vi "SDCP SMF Receiver and Trasmitter - Live Plot - Backup.vi"() -> ()   [LabVIEW 2020]
uses:
  Typedefs/SDCP - Standard Message Frame Parameters - FGV - commands.ctl
  Typedefs/SDCP - Serial Port Control - Commands.ctl
panel:
  out "Active Plot Names":string[](array[string])
  out "Value":dbl
  out "Time (ms)":dbl
  in  "Cursor Parameter":string(combo)
  out "Instantaeneous data":T1(array[cluster])
  in  "Time span (ms)":dbl
  in  "Channel 8 enable":bool
  in  "Channel 7 enable":bool
  in  "Channel 6 enable":bool
  in  "Channel 5 enable":bool
  in  "Channel 4 enable":bool
  in  "Channel 3 enable":bool
  in  "Channel 2 enable":bool
  in  "Channel 1 enable":bool
  in  "Channel 8 parameter":string(combo)
  in  "Channel 7 parameter":string(combo)
  in  "Channel 6 parameter":string(combo)
  in  "Channel 5 parameter":string(combo)
  in  "Channel 4 parameter":string(combo)
  in  "Channel 3 parameter":string(combo)
  in  "Channel 2 parameter":string(combo)
  in  "Channel 1 parameter":string(combo)
  in  "Plot file path":path
  out "Live Plot":T2(graph)
  out "Time (ms)":u32
  in  "Stop Application":bool
  in  "Trace file path":path
  in  "Baud rate":u32=9600
  in  "COM Port":refnum<visa-resource-name>
  in  "Parameter file path":path=path "E:/Projects/System Diagnostics and Control Protocol/SDCP_LabVIEW/Parameter Files/Motion_Processing.param"
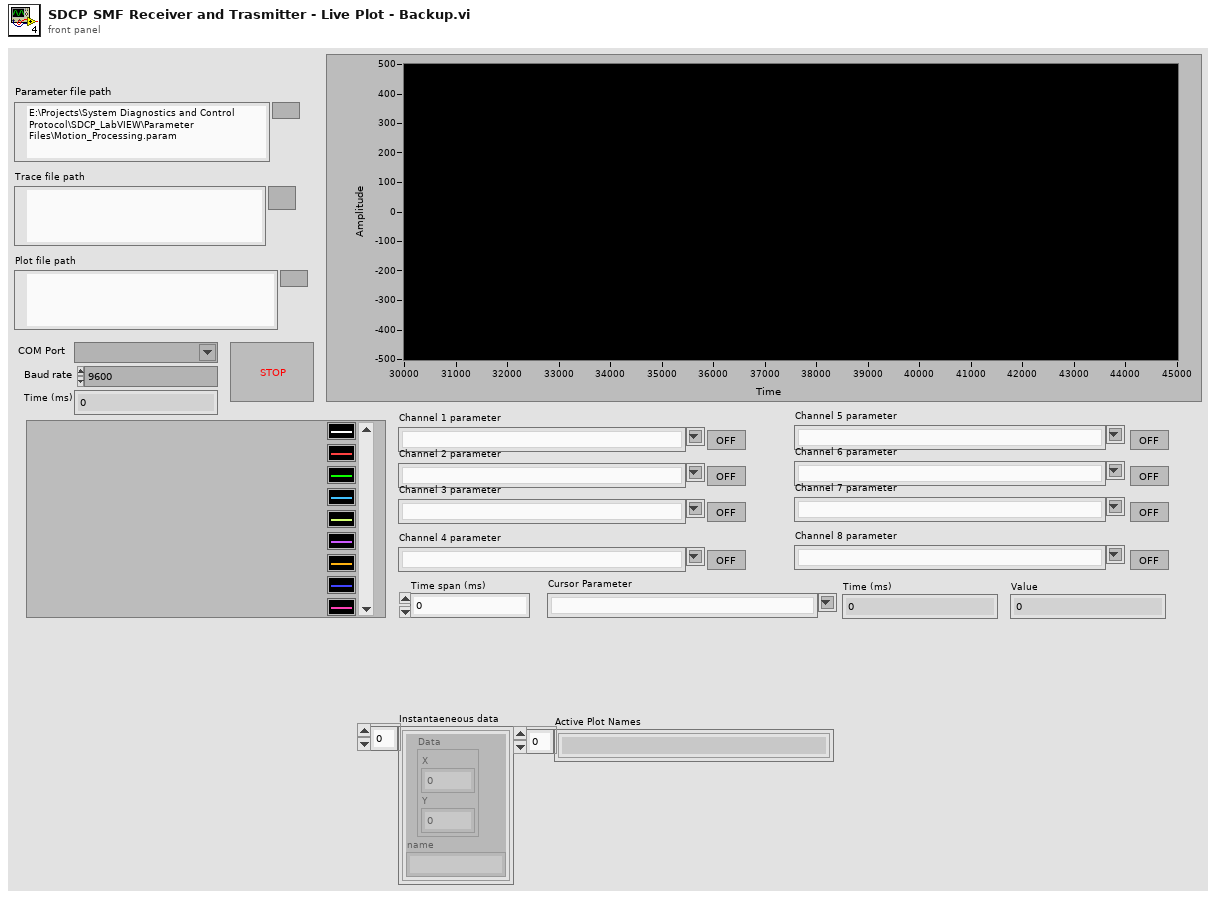
[diagram p1: front panel]
types:
  T1 = cluster{"Data":cluster{"X":dbl, "Y":dbl}, "name":string}[]
  T2 = cluster{"Plot data":cluster{"X":dbl, "Y":dbl}[]}[]
  T3 = typedef "SDCP - Serial Port Control - Commands.ctl" = enum16{"Open", "Read", "Write", "Get instance", "Close"}
  T4 = cluster{"data bytes":u8[], "Time (ms)":u32, "Direction":string}
  T5 = typedef "SDCP - Standard Message Frame Parameters - FGV - commands.ctl" = enum16{"Write descriptors", "Read descriptors", "Read values", "Load parameters from file", "Write values", "Read all descriptors"}
  T6 = typedef "SDCP - SMF parameter descriptors.ctl" = cluster{"Frame name":string, "Frame ID":i32, "Data type":string, "Start Position":i32, "Length":i32, "Factor":dbl, "Offset":dbl, "Parameter name":string, "Value":string}
  T7 = cluster{"name":string, "Data":cluster{"X":dbl, "Y":dbl}[]}
  T8 = cluster{"name":string, "Data":cluster{"X":dbl, "Y":dbl}[]}[]
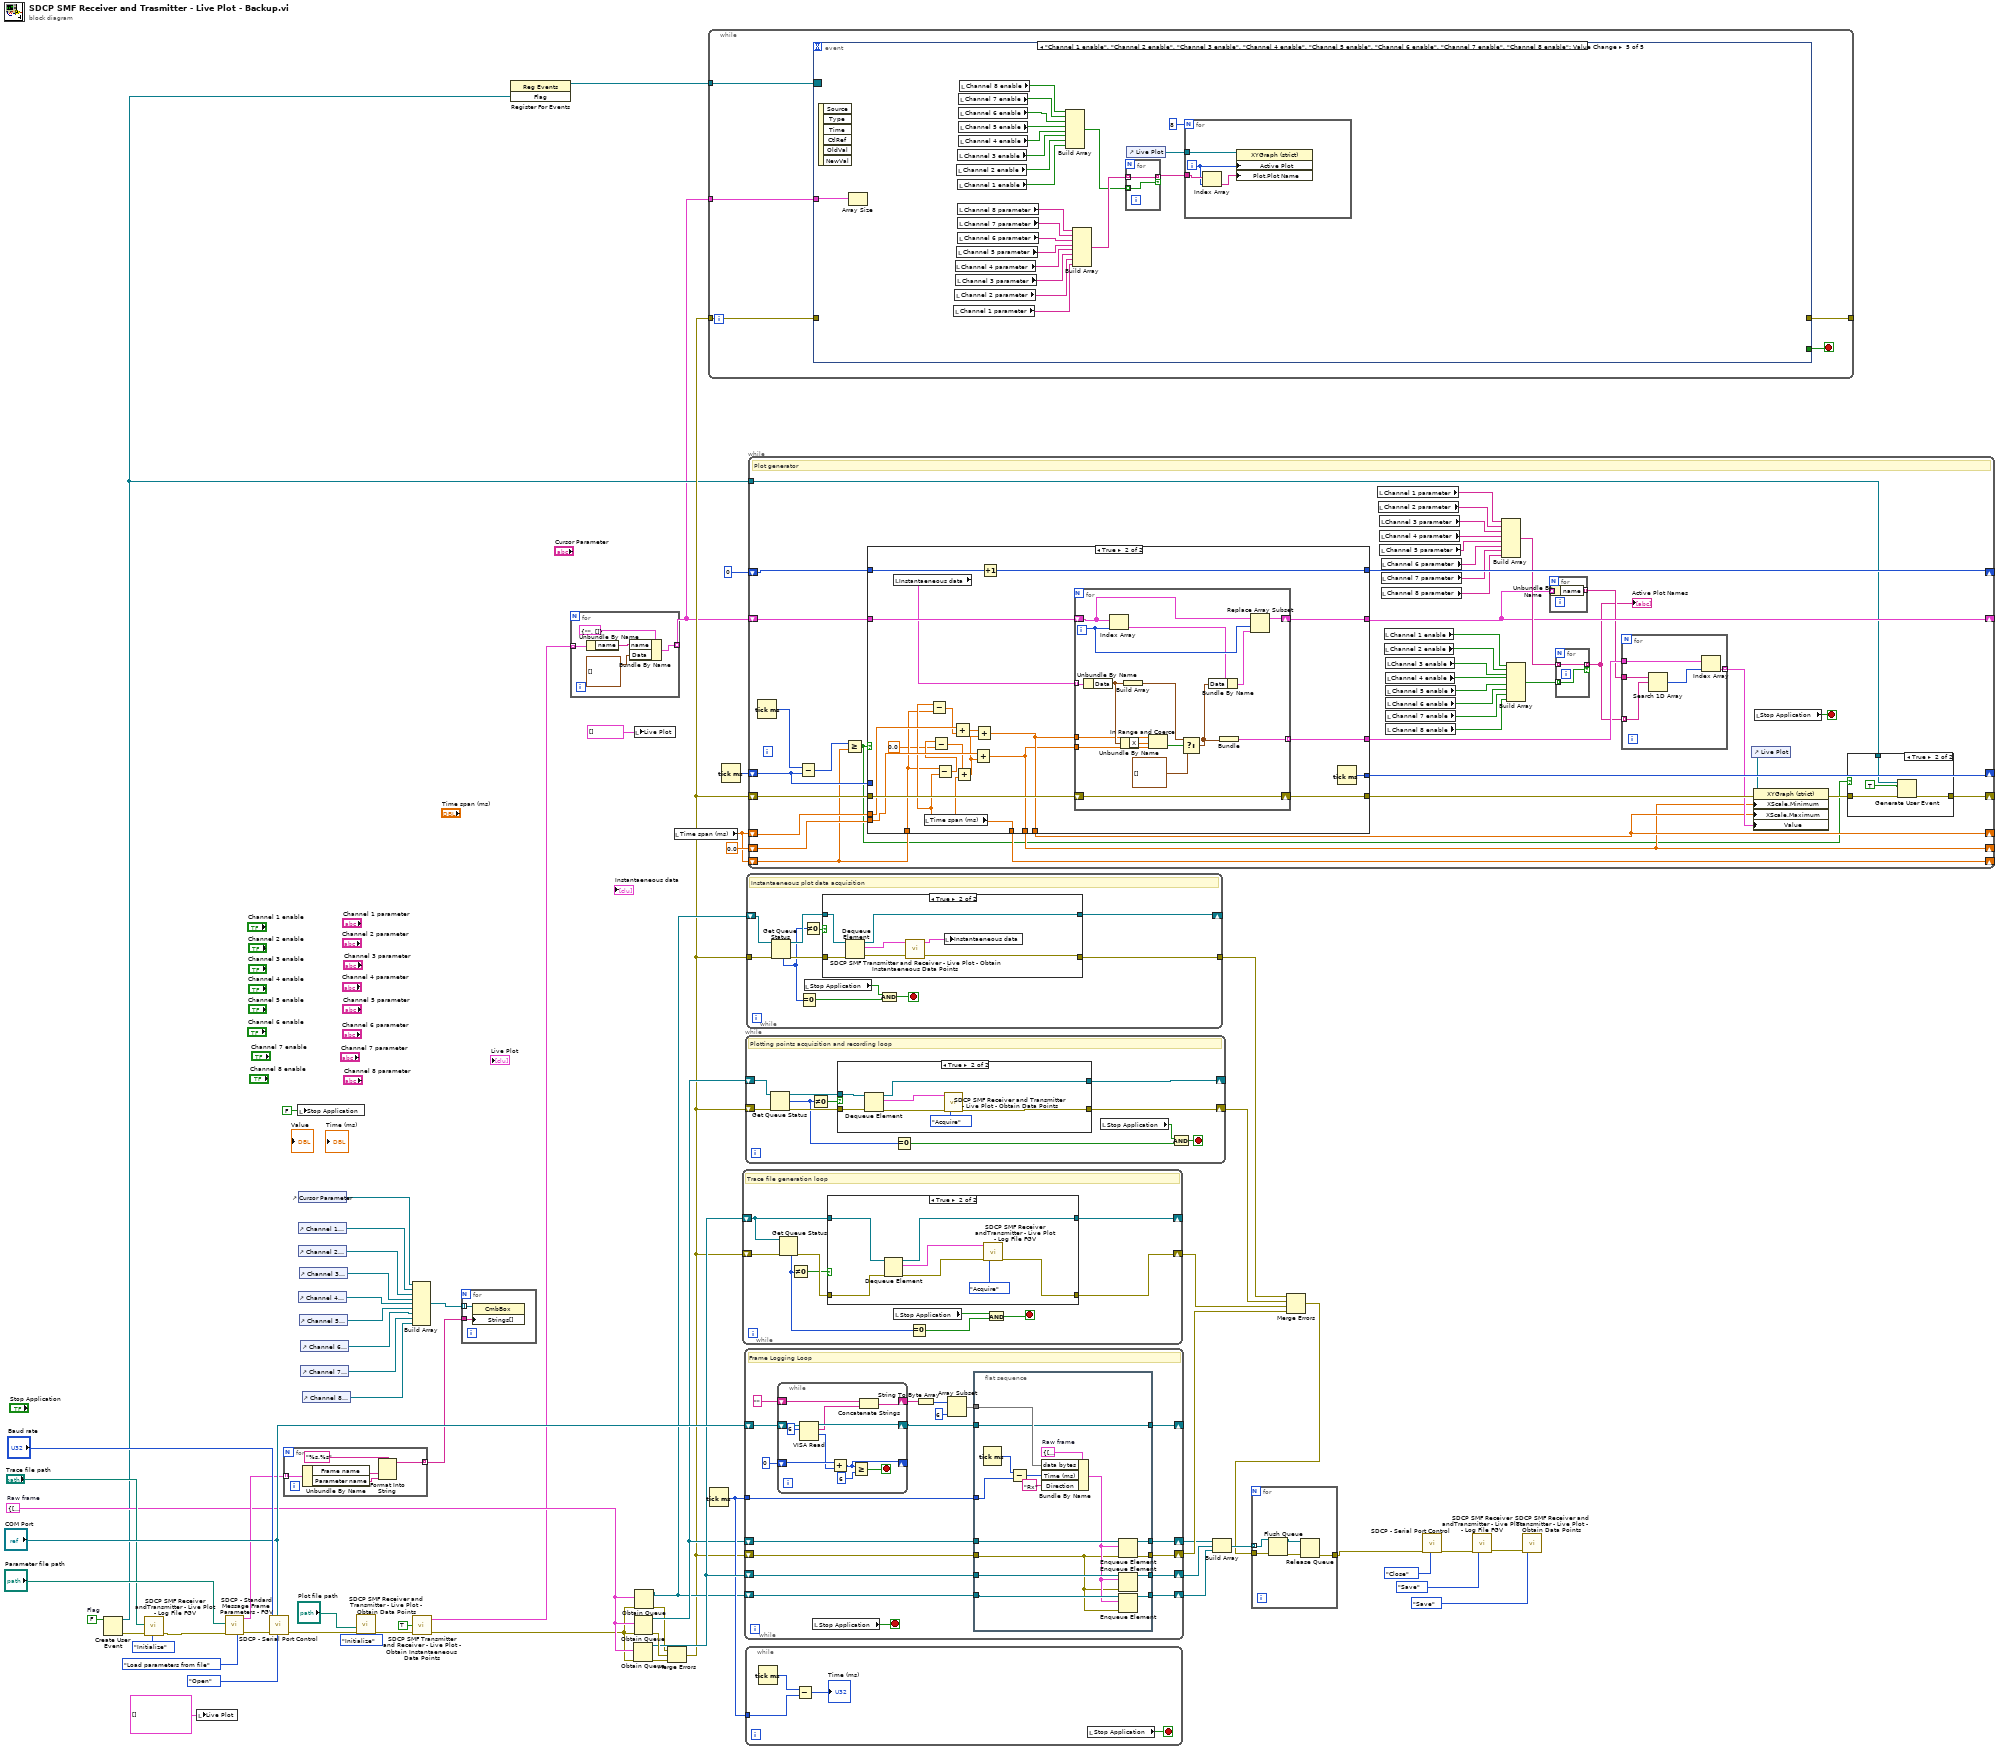
[diagram p0: block diagram]
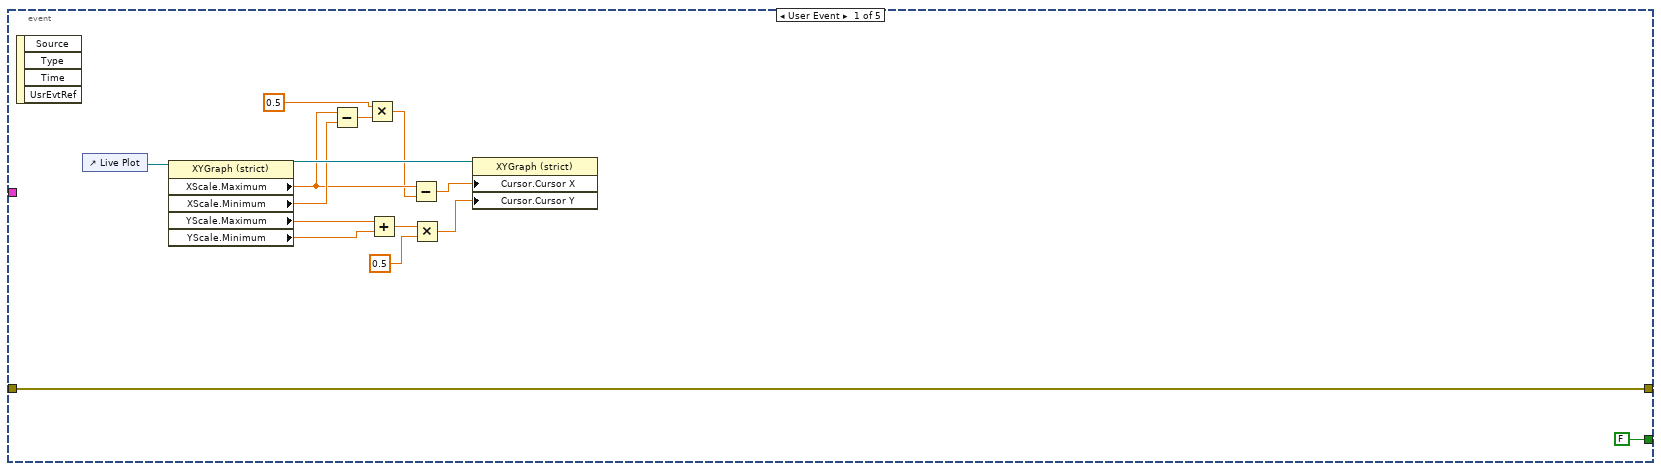
[diagram p2: hidden frame]
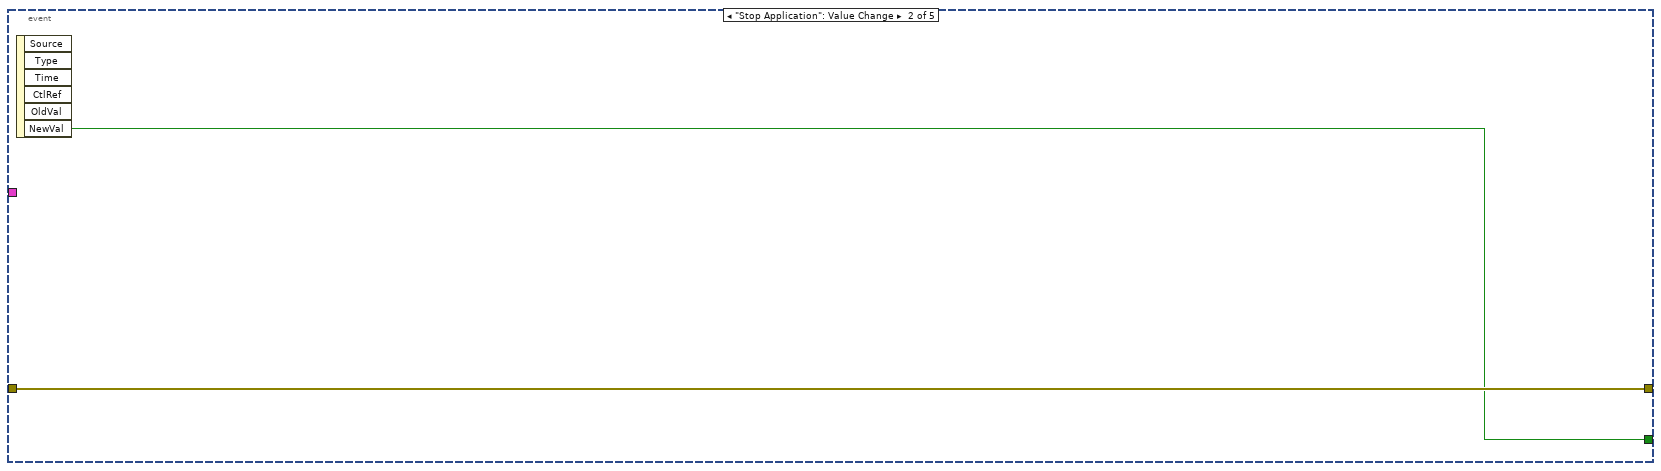
[diagram p3: hidden frame]
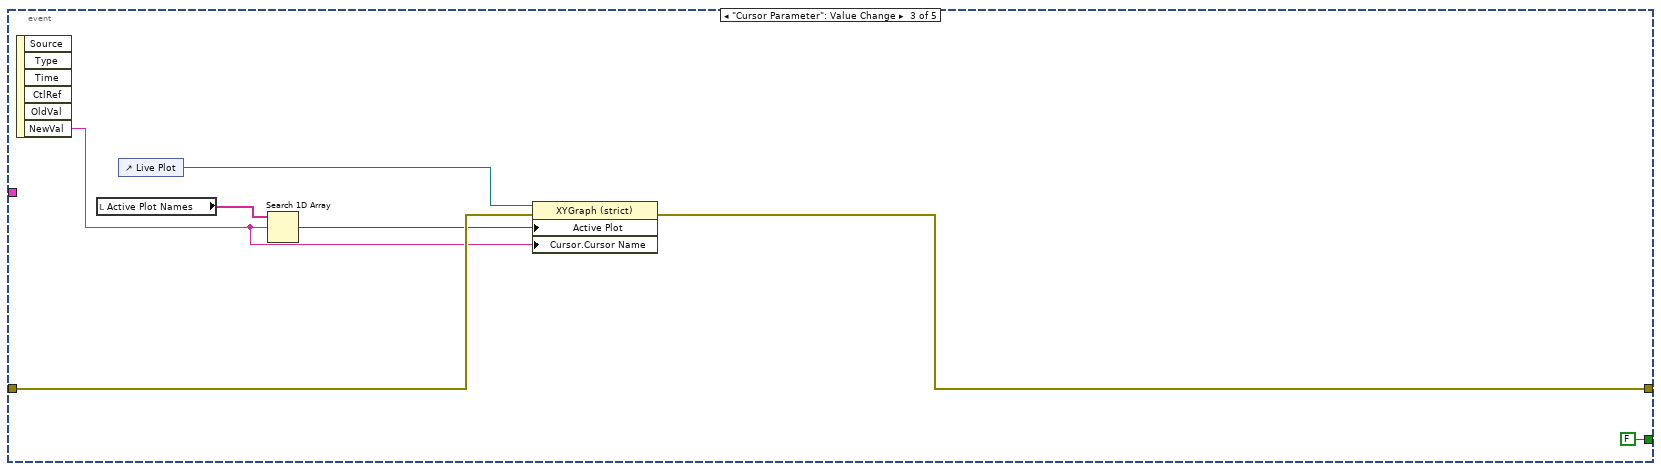
[diagram p4: hidden frame]
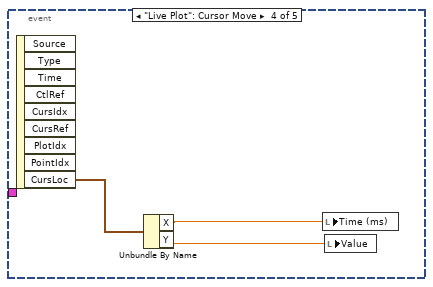
[diagram p5: hidden frame]
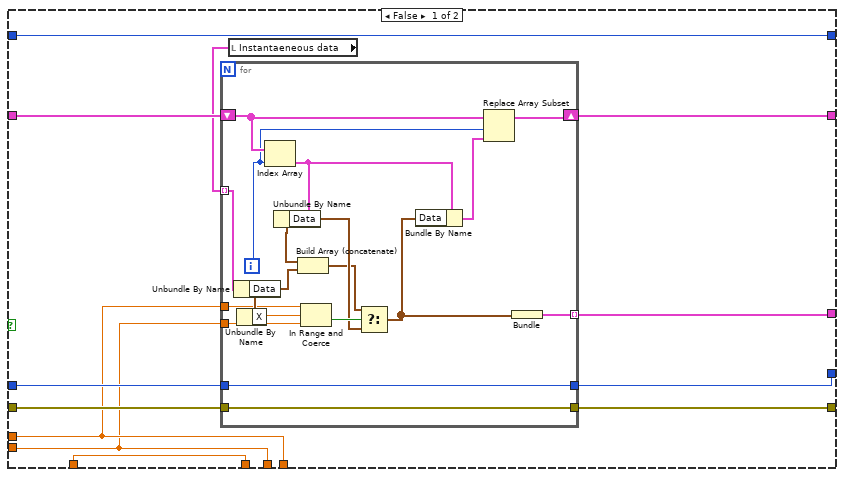
[diagram p7: hidden frame]
diagram:
  w4 = FALSE  # Flag
  w28 = T4 {"data bytes"=[], "Time (ms)"=0, "Direction"=""}  # Raw frame
  n1 = Create User Event(user event datatype=w4) -> (user event=w2:refnum<user-event>, error out=w5:errorcluster)  [unwired: 1 in]
  n2 = call "SDCP SMF Receiver andTransmitter - Live Plot - Log File FGV.vi"("error in (no error)"=w5, "Command"=enum16{"Initialize", "Acquire", "Save"}."Initialize", "Trace file path"="Trace file path") -> ("error out"=w46:errorcluster)  [unwired: 4 in]
  n3 = local write "Live Plot"(T2 [] ("Live Plot")) -> ()
  n4 = call "SDCP - Standard Message Frame Parameters - FGV.vi"("Parameter file path"="Parameter file path", "error in (no error)"=w46, "Command"=SDCP_-_Standard_Message_Frame_Parameters_-_FGV_-_commands."Load parameters from file") -> ("SMF Parameters descriptors out"=w41:T6[], "error out"=w62:errorcluster)  [unwired: 4 in]
  n5 = call "SDCP - Serial Port Control.vi"("Command"=SDCP_-_Serial_Port_Control_-_Commands."Open", "VISA resource name"="COM Port", "error in (no error)"=w62, "Baud rate"="Baud rate") -> ("error out"=w30:errorcluster)  [unwired: 4 in, 3 out]
  n6 = for {
    tunnel: w41 -> [w69] mode=indexing
    tunnel: [w65] -> w31 mode=indexing
    n7 = Unbundle By Name(w69) -> ("Frame name"=w67:string, "Parameter name"=w66:string)
    n8 = Format Into String(format string="%s.%s", w67, w66) -> (resulting string=w65:string)  [unwired: 2 in, 1 out]
  }
  n9 = local write "Stop Application"(FALSE ("Stop Application")) -> ()
  n10 = control-ref of="Cursor Parameter"() -> (w7:refnum<vi>)
  n11 = control-ref of="Channel 1 parameter"() -> (w40:refnum<vi>)
  n12 = control-ref of="Channel 2 parameter"() -> (w39:refnum<vi>)
  n13 = control-ref of="Channel 4 parameter"() -> (w37:refnum<vi>)
  n14 = control-ref of="Channel 3 parameter"() -> (w38:refnum<vi>)
  n15 = control-ref of="Channel 5 parameter"() -> (w36:refnum<vi>)
  n16 = control-ref of="Channel 6 parameter"() -> (w35:refnum<vi>)
  n17 = control-ref of="Channel 7 parameter"() -> (w34:refnum<vi>)
  n18 = control-ref of="Channel 8 parameter"() -> (w33:refnum<vi>)
  n19 = call "SDCP SMF Receiver and Transmitter - Live Plot - Obtain Data Points.vi"("error in (no error)"=w30, "Plot file path"="Plot file path", "Command"=enum16{"Initialize", "Acquire", "Save"}."Initialize") -> ("error out"=w17:errorcluster)  [unwired: 4 in]
  n20 = Build Array(w7, w40, w39, w38, w37, w36, w35, w34, w33) -> (w32:refnum<vi>[])
  n21 = call "SDCP SMF Transmitter and Receiver - Live Plot - Obtain Instantaeneous Data Points.vi"("error in (no error)"=w17, "Initialize ?"=TRUE) -> ("error out"=w16:errorcluster, "Instantaeneous data"=w13:T1)  [unwired: 2 in]
  n22 = for {
    tunnel: w32 -> [w71] mode=indexing
    tunnel: w31 -> [w70]
    n23 = property class="CmbBox"(reference=w71, "Strings[]"=w70) -> ()  [unwired: 1 in, 2 out]
  }
  n24 = register-events(w2) -> (reference out=w3:refnum<event-registration>)  [unwired: 2 in, 1 out]
  n25 = for {
    tunnel: w13 -> [w76] mode=indexing
    tunnel: [w73] -> w1 mode=indexing
    n26 = Unbundle By Name(w76) -> ("name"=w74:string)
    n27 = Bundle By Name(cluster=T7 {"name"="", "Data"=[]}, "name"=w74, "Data"=cluster{"X":dbl, "Y":dbl}[] []) -> (w73:T7)
  }
  n28 = Obtain Queue(element data type=w28, error in (no error)=w16) -> (queue out=w56:refnum<queue>, error out=w57:errorcluster)  [unwired: 3 in, 1 out]
  n29 = local write "Live Plot"(cluster{"Data":cluster{"X":dbl, "Y":dbl}[]}[] []) -> ()
  n30 = Obtain Queue(element data type=w28, error in (no error)=w16) -> (queue out=w47:refnum<queue>, error out=w58:errorcluster)  [unwired: 3 in, 1 out]
  n31 = Obtain Queue(element data type=w28, error in (no error)=w16) -> (queue out=w19:refnum<queue>, error out=w27:errorcluster)  [unwired: 3 in, 1 out]
  n32 = Merge Errors(w27, w58, w57) -> (w6:errorcluster)
  n33 = local read "Time span (ms)"() -> (w8:dbl)
  n34 = while {
    tunnel: w6 -> [w81]
    tunnel: [w80] -> _
    tunnel: w3 -> [w78]
    tunnel: w1 -> [w77]
    stop <- w79 stop-if-true
    n35 = event shown="[4] \"Channel 1 enable\", \"Channel 2 enable\", \"Channel 3 enable\", \"Channel 4 enable\", \"Channel 5 enable\", \"Channel 6 enable\", \"Channel 7 enable\", \"Channel 8 enable\": Value Change" {
      selector: w78 -> [_ _ _ _ _]
      dyn-events: _ -> [_ _ _ _ _]
      timeout: _ -> [_ _ _ _ _]
      tunnel: w81 -> [w96 w98 w104 _ _]
      tunnel: [w96 w98 w100 _ _] -> w80
      tunnel: [FALSE w97 FALSE ("NewVal") _ _] -> w79
      tunnel: w77 -> [_ _ _ _ w110]
      event User Event {
        n36 = event-data() -> ()  [unwired: 1 in, 4 out]
        n37 = control-ref of="Live Plot"() -> (w94:refnum<vi>)
        n38 = property class="XYGraph (strict)"(reference=w94) -> (reference out=w89:refnum<vi>, "XScale.Maximum"=w86:dbl, "XScale.Minimum"=w87:dbl, "YScale.Maximum"=w93:dbl, "YScale.Minimum"=w92:dbl)  [unwired: 1 in, 1 out]
        n39 = Subtract(x=w86, y=w87) -> (x-y=w85:dbl)
        n40 = Multiply(x=0.5, y=w85) -> (x*y=w83:dbl)
        n41 = Add(x=w93, y=w92) -> (x+y=w91:dbl)
        n42 = Subtract(x=w86, y=w83) -> (x-y=w82:dbl)
        n43 = Multiply(x=w91, y=0.5) -> (x*y=w88:dbl)
        n44 = property class="XYGraph (strict)"(reference=w89, "Cursor.Cursor X"=w82, "Cursor.Cursor Y"=w88) -> ()  [unwired: 1 in, 2 out]
      }
      event "Stop Application": Value Change {
        n45 = event-data() -> ("NewVal"=w97:bool)  [unwired: 1 in, 5 out]
      }
      event "Cursor Parameter": Value Change {
        n46 = event-data() -> ("NewVal"=w101:string)  [unwired: 1 in, 5 out]
        n47 = local read "Active Plot Names"() -> (w99:string[])
        n48 = control-ref of="Live Plot"() -> (w103:refnum<vi>)
        n49 = Search 1D Array(1D array=w99, element=w101) -> (index of element=w102:i32)  [unwired: 1 in]
        n50 = property class="XYGraph (strict)"(reference=w103, error in=w104, "Active Plot"=w102, "Cursor.Cursor Name"=w101) -> (error out=w100:errorcluster)  [unwired: 1 out]
      }
      event "Live Plot": Cursor Move {
        n51 = event-data() -> ("CursLoc"=w108:cluster{"X":dbl, "Y":dbl})  [unwired: 1 in, 8 out]
        n52 = Unbundle By Name(w108) -> ("X"=w107:dbl, "Y"=w106:dbl)
        n53 = local write "Time (ms)"(w107) -> ()
        n54 = local write "Value"(w106) -> ()
      }
      event "Channel 1 enable", "Channel 2 enable", "Channel 3 enable", "Channel 4 enable", "Channel 5 enable", "Channel 6 enable", "Channel 7 enable", "Channel 8 enable": Value Change {
        n55 = event-data() -> ()  [unwired: 1 in, 6 out]
        n56 = Array Size(array=w110) -> ()  [unwired: 1 out]
        n57 = local read "Channel 1 parameter"() -> (w115:string)
        n58 = local read "Channel 2 parameter"() -> (w116:string)
        n59 = local read "Channel 4 parameter"() -> (w118:string)
        n60 = local read "Channel 3 parameter"() -> (w117:string)
        n61 = local read "Channel 2 enable"() -> (w124:bool)
        n62 = local read "Channel 5 parameter"() -> (w119:string)
        n63 = local read "Channel 3 enable"() -> (w125:bool)
        n64 = local read "Channel 1 enable"() -> (w123:bool)
        n65 = local read "Channel 8 parameter"() -> (w122:string)
        n66 = local read "Channel 7 parameter"() -> (w121:string)
        n67 = local read "Channel 6 parameter"() -> (w120:string)
        n68 = local read "Channel 7 enable"() -> (w129:bool)
        n69 = local read "Channel 6 enable"() -> (w128:bool)
        n70 = local read "Channel 5 enable"() -> (w127:bool)
        n71 = local read "Channel 4 enable"() -> (w126:bool)
        n72 = local read "Channel 8 enable"() -> (w130:bool)
        n73 = Build Array(w130, w129, w128, w127, w126, w125, w124, w123) -> (w113:bool[])
        n74 = Build Array(w122, w121, w120, w119, w118, w117, w116, w115) -> (w114:string[])
        n75 = for {
          tunnel: w114 -> [w136] mode=indexing
          tunnel: w113 -> [w135] mode=indexing
          tunnel: [w136] -> w111 mode=indexing if=w135
        }
        n76 = control-ref of="Live Plot"() -> (w112:refnum<vi>)
        n77 = for {
          N: 8 -> [_]
          tunnel: w112 -> [w134]
          tunnel: w111 -> [w133]
          i -> [w132]
          n78 = Index Array(array=w133, index=w132) -> (element=w131:string)
          n79 = property class="XYGraph (strict)"(reference=w134, "Active Plot"=w132, "Plot.Plot Name"=w131) -> ()  [unwired: 1 in, 2 out]
        }
      }
    }
  }
  n80 = Tick Count (ms)() -> (millisecond timer value=w48:u32)
  n81 = Tick Count (ms)() -> (millisecond timer value=w14:u32)
  n82 = while {
    shift-right: [w144] -> w50
    shift-left: w6 -> [w146]
    shift-right: [w143] -> _
    shift-left: w56 -> [w145]
    stop <- w139 stop-if-true
    # "Trace file generation loop"
    n83 = Get Queue Status(queue=w145, error in (no error)=w146) -> (error out=w142:errorcluster, # elements in queue=w138:i32)  [unwired: 1 in, 6 out]
    n84 = Not Equal To 0?(x=w138) -> (x != 0?=w141:bool)
    n85 = case shown="True" w141 {
      tunnel: w142 -> [w148 w153]
      tunnel: [w148 w155] -> w144
      tunnel: w145 -> [w147 w151]
      tunnel: [w147 w150] -> w143
      frame False {
      }
      frame True {
        n86 = Dequeue Element(queue=w151, error in (no error)=w153) -> (queue out=w150:refnum<queue>, element=w149:T4, error out=w152:errorcluster)  [unwired: 1 in, 1 out]
        n87 = call "SDCP SMF Receiver andTransmitter - Live Plot - Log File FGV.vi"("error in (no error)"=w152, "Command"=enum16{"Initialize", "Acquire", "Save"}."Acquire", "Raw frame"=w149) -> ("error out"=w155:errorcluster)  [unwired: 4 in]
      }
    }
    n88 = local read "Stop Application"() -> (w140:bool)
    n89 = Equal To 0?(x=w138) -> (x = 0?=w137:bool)
    n90 = And(x=w140, y=w137) -> (x .and. y?=w139:bool)
  }
  n91 = while {
    tunnel: w48 -> [w167]
    shift-right: [w163] -> _
    shift-left: "COM Port" -> [w174]
    shift-right: [w165] -> w49
    shift-left: w6 -> [w166]
    shift-right: [w161] -> w25
    shift-left: w47 -> [w162]
    shift-right: [w159] -> w24
    shift-left: w56 -> [w160]
    shift-right: [w156] -> w23
    shift-left: w19 -> [w157]
    stop <- w158 stop-if-true
    # "Frame Logging Loop"
    n92 = while {
      shift-right: [w200] -> w164
      shift-left: w174 -> [w201]
      shift-right: [w192] -> w171
      shift-left: "" -> [w194]
      shift-right: [w196] -> _
      shift-left: 0 -> [w199]
      stop <- w195 stop-if-true
      n93 = VISA Read(VISA resource name=w201, byte count=u32 6) -> (VISA resource name out=w200:refnum<visa-resource-name>, read buffer=w193:string, return count=w198:u32)  [unwired: 1 in, 1 out]
      n94 = Add(x=w199, y=w198) -> (x+y=w196:u32)
      n95 = Greater Or Equal?(x=w196, y=u32 6) -> (x >= y?=w195:bool)
      n96 = Concatenate Strings(w194, w193) -> (w192:string)
    }
    n97 = local read "Stop Application"() -> (w158:bool)
    n98 = String To Byte Array(string=w171) -> (unsigned byte array=w170:u8[])
    n99 = Array Subset(array=w170, length=6) -> (w168:u8[])  [unwired: 1 in]
    n100 = flat-sequence {
      tunnel: w168 -> [w180]
      tunnel: w167 -> [w189]
      tunnel: w166 -> [w175]
      tunnel: [w186] -> w165
      tunnel: w164 -> [w179]
      tunnel: [w179] -> w163
      tunnel: w162 -> [w185]
      tunnel: [w184] -> w161
      tunnel: w160 -> [w183]
      tunnel: [w182] -> w159
      tunnel: w157 -> [w178]
      tunnel: [w176] -> w156
      frame #0 {
        w188 = T4 {"data bytes"=[], "Time (ms)"=0, "Direction"=""}  # Raw frame
        n101 = Tick Count (ms)() -> (millisecond timer value=w190:u32)
        n102 = Subtract(x=w190, y=w189) -> (x-y=w187:u32)
        n103 = Bundle By Name(cluster=w188, "data bytes"=w180, "Time (ms)"=w187, "Direction"="Rx") -> (w177:T4)
        n104 = Enqueue Element(queue=w185, element=w177, error in (no error)=w175) -> (queue out=w184:refnum<queue>, error out=w186:errorcluster)  [unwired: 1 in, 1 out]
        n105 = Enqueue Element(queue=w183, element=w177, error in (no error)=w175) -> (queue out=w182:refnum<queue>)  [unwired: 1 in, 2 out]
        n106 = Enqueue Element(queue=w178, element=w177, error in (no error)=w175) -> (queue out=w176:refnum<queue>)  [unwired: 1 in, 2 out]
      }
    }
  }
  n107 = while {
    shift-right: [w206] -> _
    shift-left: w47 -> [w211]
    shift-right: [w208] -> w26
    shift-left: w6 -> [w212]
    stop <- w204 stop-if-true
    # "Plotting points acquisition and recording loop"
    n108 = Get Queue Status(queue=w211, error in (no error)=w212) -> (queue out=w207:refnum<queue>, error out=w209:errorcluster, # elements in queue=w205:i32)  [unwired: 1 in, 5 out]
    n109 = Not Equal To 0?(x=w205) -> (x != 0?=w210:bool)
    n110 = case shown="True" w210 {
      tunnel: w209 -> [w214 w221]
      tunnel: [w214 w216] -> w208
      tunnel: w207 -> [w213 w220]
      tunnel: [w213 w219] -> w206
      frame False {
      }
      frame True {
        n111 = Dequeue Element(queue=w220, error in (no error)=w221) -> (queue out=w219:refnum<queue>, element=w217:T4, error out=w218:errorcluster)  [unwired: 1 in, 1 out]
        n112 = call "SDCP SMF Receiver and Transmitter - Live Plot - Obtain Data Points.vi"("error in (no error)"=w218, "Command"=enum16{"Initialize", "Acquire", "Save"}."Acquire", "Raw frame"=w217) -> ("error out"=w216:errorcluster)  [unwired: 4 in]
      }
    }
    n113 = Equal To 0?(x=w205) -> (x = 0?=w202:bool)
    n114 = local read "Stop Application"() -> (w203:bool)
    n115 = And(x=w203, y=w202) -> (x .and. y?=w204:bool)
  }
  n116 = while {
    tunnel: w48 -> [w224]
    stop <- w222 stop-if-true
    n117 = Tick Count (ms)() -> (millisecond timer value=w225:u32)
    n118 = Subtract(x=w225, y=w224) -> (x-y=→"Time (ms)":u32)
    n119 = local read "Stop Application"() -> (w222:bool)
  }
  n120 = while {
    shift-right: [w228] -> _
    shift-left: w19 -> [w235]
    tunnel: w6 -> [w236]
    tunnel: [w227] -> w18
    stop <- w231 stop-if-true
    # "Instantaeneous plot data acquisition"
    n121 = Get Queue Status(queue=w235, error in (no error)=w236) -> (queue out=w229:refnum<queue>, error out=w230:errorcluster, # elements in queue=w226:i32)  [unwired: 1 in, 5 out]
    n122 = Equal To 0?(x=w226) -> (x = 0?=w233:bool)
    n123 = Not Equal To 0?(x=w226) -> (x != 0?=w234:bool)
    n124 = local read "Stop Application"() -> (w232:bool)
    n125 = case shown="True" w234 {
      tunnel: w230 -> [w237 w245]
      tunnel: w229 -> [w238 w244]
      tunnel: [w238 w243] -> w228
      tunnel: [w237 w240] -> w227
      frame False {
      }
      frame True {
        n126 = Dequeue Element(queue=w244, error in (no error)=w245) -> (queue out=w243:refnum<queue>, element=w241:T4, error out=w242:errorcluster)  [unwired: 1 in, 1 out]
        n127 = call "SDCP SMF Transmitter and Receiver - Live Plot - Obtain Instantaeneous Data Points.vi"("error in (no error)"=w242, "Raw frame"=w241) -> ("error out"=w240:errorcluster, "Instantaeneous data"=w239:T1)  [unwired: 2 in]
        n128 = local write "Instantaeneous data"(w239) -> ()
      }
    }
    n129 = And(x=w232, y=w233) -> (x .and. y?=w231:bool)
  }
  n130 = while {
    shift-right: [w249] -> _
    shift-left: w6 -> [w286]
    shift-right: [w285] -> _
    shift-left: w14 -> [w283]
    shift-right: [w258] -> _
    shift-left: w1 -> [w284]
    shift-right: [w282] -> _
    shift-left: 0 -> [w281]
    shift-right: [w256] -> _
    shift-left: w8 -> [w255]
    shift-right: [w253] -> _
    shift-left: 0.0 -> [w254]
    shift-right: [w252] -> _
    shift-left: w8 -> [w251]
    tunnel: w2 -> [w248]
    stop <- w289 stop-if-true
    # "Plot generator"
    n131 = Tick Count (ms)() -> (millisecond timer value=w288:u32)
    n132 = Subtract(x=w288, y=w283) -> (x-y=w287:u32)
    n133 = Greater Or Equal?(x=w287, y=w251) -> (x >= y?=w247:bool)
    n134 = case shown="True" w247 {
      tunnel: w286 -> [w310 w348]
      tunnel: [w309 w349] -> w280
      tunnel: [w312 w353] -> w285
      tunnel: w284 -> [w315 w352]
      tunnel: [w311 w350] -> w258
      tunnel: w283 -> [w313 _]
      tunnel: [w307 w347] -> w260
      tunnel: w281 -> [w308 w346]
      tunnel: [w308 w345] -> w282
      tunnel: [w306 w342] -> w256
      tunnel: [w305 w341] -> w253
      tunnel: w255 -> [w306 w344]
      tunnel: w254 -> [w305 w343]
      tunnel: [w304 w339] -> w252
      tunnel: w251 -> [w304 w338]
      frame False {
        n135 = local read "Instantaeneous data"() -> (w314:T1)
        n136 = for {
          shift-right: [w327] -> w311
          shift-left: w315 -> [w330]
          tunnel: w314 -> [w331] mode=indexing
          tunnel: w313 -> [w326]
          tunnel: [w326] -> w312
          tunnel: w310 -> [w325]
          tunnel: [w325] -> w309
          tunnel: [w324] -> w307 mode=indexing
          tunnel: w306 -> [w317]
          tunnel: w305 -> [w316]
          i -> [w329]
          n137 = Unbundle By Name(w331) -> ("Data"=w320:cluster{"X":dbl, "Y":dbl})
          n138 = Unbundle By Name(w320) -> ("X"=w323:dbl)
          n139 = Index Array(array=w330, index=w329) -> (element=w332:T7)
          n140 = Unbundle By Name(w332) -> ("Data"=w321:cluster{"X":dbl, "Y":dbl}[])
          n141 = Build Array (concatenate)(w321, w320) -> (w319:cluster{"X":dbl, "Y":dbl}[])
          n142 = In Range and Coerce(upper limit=w317, x=w323, lower limit=w316) -> (In Range?=w322:bool)  [unwired: 1 out]
          n143 = Select(t=w319, s=w322, f=w321) -> (s? t:f=w318:cluster{"X":dbl, "Y":dbl}[])
          n144 = Bundle By Name(cluster=w332, "Data"=w318) -> (w328:T7)
          n145 = Replace Array Subset(array=w330, new element=w328, index=w329) -> (w327:T8)
          n146 = Bundle("Data"=w318) -> (w324:cluster{"Data":cluster{"X":dbl, "Y":dbl}[]})  [unwired: 1 in]
        }
      }
      frame True {
        n147 = local read "Instantaeneous data"() -> (w351:T1)
        n148 = local read "Time span (ms)"() -> (w339:dbl)
        n149 = Subtract(x=w339, y=w338) -> (x-y=w336:dbl)
        n150 = Subtract(x=w338, y=w339) -> (x-y=w335:dbl)
        n151 = Subtract(x=w335, y=0.0) -> (x-y=w334:dbl)
        n152 = Add(x=w344, y=w336) -> (x+y=w337:dbl)
        n153 = Add(x=w334, y=w339) -> (x+y=w340:dbl)
        n154 = Add(x=w343, y=w340) -> (x+y=w341:dbl)
        n155 = Add(x=w337, y=w340) -> (x+y=w342:dbl)
        n156 = Increment(x=w346) -> (x+1=w345:i32)
        n157 = for {
          shift-right: [w360] -> w350
          shift-left: w352 -> [w369]
          tunnel: w351 -> [w367] mode=indexing
          shift-right: [w364] -> w349
          shift-left: w348 -> [w364]
          tunnel: [w363] -> w347 mode=indexing
          tunnel: w342 -> [w355]
          tunnel: w341 -> [w354]
          i -> [w368]
          n158 = Unbundle By Name(w367) -> ("Data"=w362:cluster{"X":dbl, "Y":dbl})
          n159 = Index Array(array=w369, index=w368) -> (element=w366:T7)
          n160 = Unbundle By Name(w362) -> ("X"=w361:dbl)
          n161 = Build Array(w362) -> (w358:cluster{"X":dbl, "Y":dbl}[])
          n162 = In Range and Coerce(upper limit=w355, x=w361, lower limit=w354) -> (In Range?=w359:bool)  [unwired: 1 out]
          n163 = Select(t=w358, s=w359, f=cluster{"X":dbl, "Y":dbl}[] []) -> (s? t:f=w357:cluster{"X":dbl, "Y":dbl}[])
          n164 = Bundle By Name(cluster=w366, "Data"=w357) -> (w365:T7)
          n165 = Bundle("f"=w357) -> (w363:cluster{"f":cluster{"X":dbl, "Y":dbl}[]})  [unwired: 1 in]
          n166 = Replace Array Subset(array=w369, new element=w365, index=w368) -> (w360:T8)
        }
        n167 = Tick Count (ms)() -> (millisecond timer value=w353:u32)
      }
    }
    n168 = local read "Channel 1 parameter"() -> (w278:string)
    n169 = local read "Channel 2 parameter"() -> (w277:string)
    n170 = local read "Channel 3 parameter"() -> (w276:string)
    n171 = local read "Channel 4 parameter"() -> (w275:string)
    n172 = local read "Channel 5 parameter"() -> (w274:string)
    n173 = local read "Channel 6 parameter"() -> (w273:string)
    n174 = local read "Channel 7 parameter"() -> (w272:string)
    n175 = local read "Channel 8 parameter"() -> (w271:string)
    n176 = local read "Channel 1 enable"() -> (w270:bool)
    n177 = local read "Channel 2 enable"() -> (w269:bool)
    n178 = local read "Channel 3 enable"() -> (w268:bool)
    n179 = local read "Channel 4 enable"() -> (w267:bool)
    n180 = local read "Channel 5 enable"() -> (w266:bool)
    n181 = local read "Channel 6 enable"() -> (w265:bool)
    n182 = local read "Channel 7 enable"() -> (w264:bool)
    n183 = local read "Channel 8 enable"() -> (w263:bool)
    n184 = Build Array(w278, w277, w276, w275, w274, w273, w272, w271) -> (w261:string[])
    n185 = Build Array(w270, w269, w268, w267, w266, w265, w264, w263) -> (w262:bool[])
    n186 = for {
      tunnel: w258 -> [w296] mode=indexing
      tunnel: [w295] -> w257 mode=indexing
      n187 = Unbundle By Name(w296) -> ("name"=w295:string)
    }
    n188 = for {
      tunnel: w262 -> [w302] mode=indexing
      tunnel: w261 -> [w303] mode=indexing
      tunnel: [w303] -> w246 mode=indexing if=w302
    }
    "Active Plot Names" <- w246
    n189 = for {
      tunnel: w246 -> [w298] mode=indexing
      tunnel: w260 -> [w301]
      tunnel: [w299] -> w259 mode=indexing
      tunnel: w257 -> [w297]
      n190 = Search 1D Array(1D array=w297, element=w298) -> (index of element=w300:i32)  [unwired: 1 in]
      n191 = Index Array(array=w301, index=w300) -> (element=w299:cluster{"f":cluster{"X":dbl, "Y":dbl}[]})
    }
    n192 = control-ref of="Live Plot"() -> (w279:refnum<vi>)
    n193 = property class="XYGraph (strict)"(reference=w279, error in=w280, "XScale.Minimum"=w253, "XScale.Maximum"=w256, "Value"=w259) -> (error out=w250:errorcluster)  [unwired: 1 out]
    n194 = local read "Stop Application"() -> (w289:bool)
    n195 = case shown="True" w247 {
      tunnel: w250 -> [w290 w294]
      tunnel: [w290 w293] -> w249
      tunnel: w248 -> [_ w291]
      frame False {
      }
      frame True {
        n196 = Generate User Event(user event=w291, event data cluster=TRUE, error in=w294) -> (error out=w293:errorcluster)  [unwired: 1 in, 1 out]
      }
    }
  }
  n197 = Build Array(w25, w24, w23) -> (w22:refnum<queue>[])
  n198 = Merge Errors(w18, w26, w50, w49) -> (w21:errorcluster)
  n199 = for {
    tunnel: w22 -> [w373] mode=indexing
    tunnel: w21 -> [w374]
    tunnel: [w370] -> w20
    n200 = Flush Queue(queue=w373, error in (no error)=w374) -> (queue out=w371:refnum<queue>, error out=w372:errorcluster)  [unwired: 1 out]
    n201 = Release Queue(queue=w371, error in (no error)=w372) -> (error out=w370:errorcluster)  [unwired: 1 in, 2 out]
  }
  n202 = call "SDCP - Serial Port Control.vi"("Command"=SDCP_-_Serial_Port_Control_-_Commands."Close", "error in (no error)"=w20) -> ("error out"=w52:errorcluster)  [unwired: 6 in, 3 out]
  n203 = call "SDCP SMF Receiver andTransmitter - Live Plot - Log File FGV.vi"("error in (no error)"=w52, "Command"=enum16{"Initialize", "Acquire", "Save"}."Save") -> ("error out"=w43:errorcluster)  [unwired: 5 in]
  n204 = call "SDCP SMF Receiver and Transmitter - Live Plot - Obtain Data Points.vi"("error in (no error)"=w43, "Command"=enum16{"Initialize", "Acquire", "Save"}."Save") -> ()  [unwired: 5 in, 1 out]
